vi "Error Check.vi"(8 "error in":errorcluster, 10 "Error Query Command":string, 11 "VISA Interface in":refnum<class "VISA Interface.lvclass">) -> (0 "error out":errorcluster, 3 "VISA Interface out":refnum<class "VISA Interface.lvclass">)   [LabVIEW 2020, in "Plugin Instrument Driver.lvlib" / "VISA Interface.lvclass"]
doc: "This VI Sets the error query command and reads the response from instrument."
uses:
  VISA Interface.lvclass
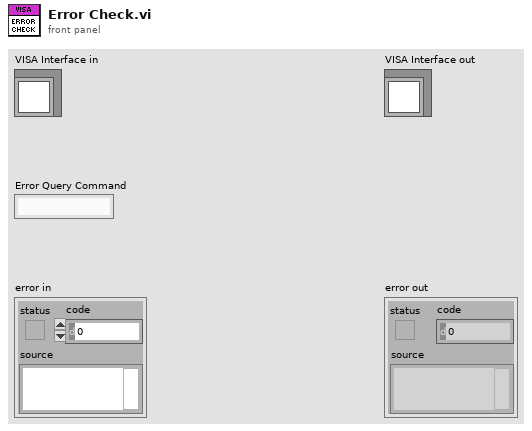
[diagram p1: front panel]
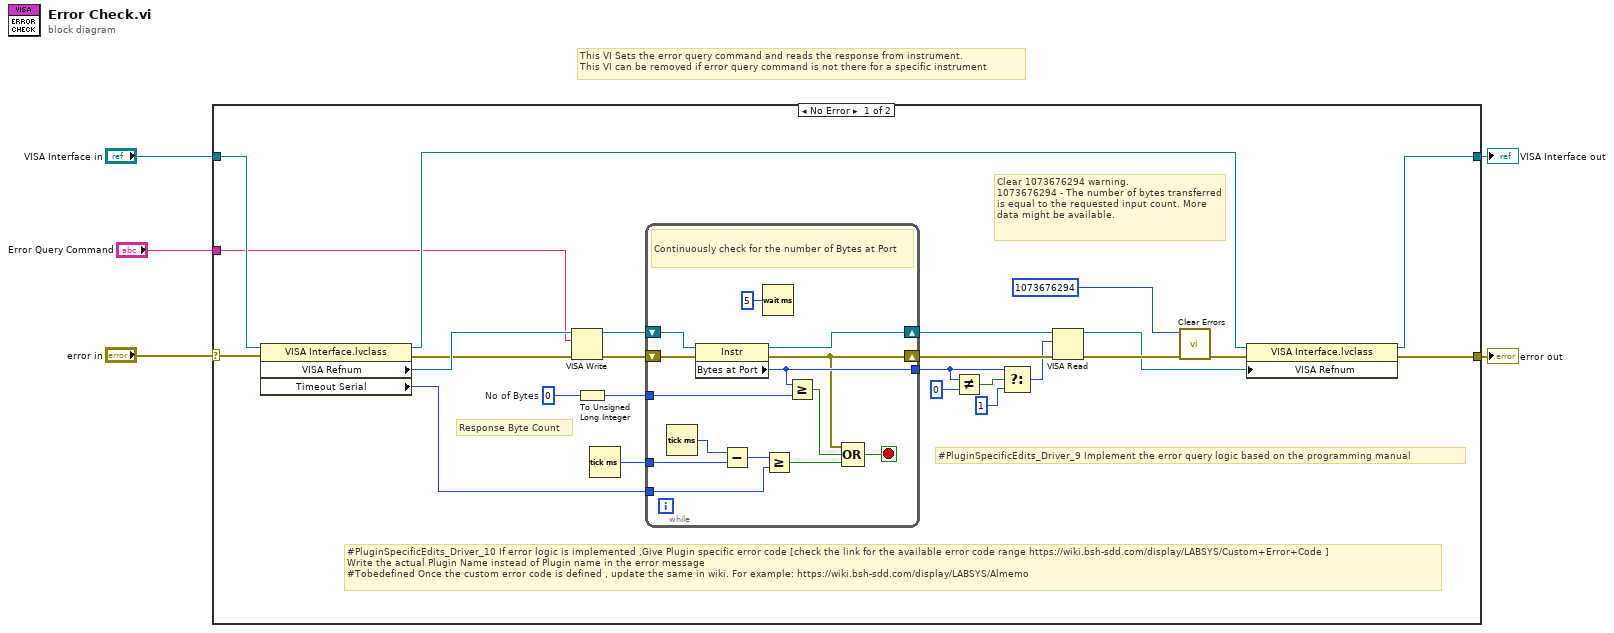
[diagram p0: block diagram]
diagram:
  # "This VI Sets the error query command and reads the response from instrument. \nThis VI can be removed if error query command is not there for a specific instrument"
  n1 = case shown="No Error" "error in" {
    selector: "error in" -> [w9 w45]
    tunnel: [w11 w46] -> w3
    tunnel: "VISA Interface in" -> [w12 w46]
    tunnel: [w10 w45] -> w2
    tunnel: "Error Query Command" -> [w6 _]
    frame No Error {
      w19 = u32 0  # No of Bytes
      # "#PluginSpecificEdits_Driver_10 If error logic is implemented ,Give Plugin specific error code [check the link for the available error code range https://wiki.bsh-sdd.com/display/LABSYS/Custom+Error+Code ]\nWrite the actual Plugin Name instead of Plugin name in the error message\n#Tobedefined Once the custom error code is defined , update the same in wiki. For example: https://wiki.bsh-sdd.com/display/LABSYS/Almemo"
      # "#PluginSpecificEdits_Driver_9 Implement the error query logic based on the programming manual"
      # "Clear 1073676294 warning.\n1073676294 - The number of bytes transferred is equal to the requested input count. More data might be available."
      # "Response Byte Count"
      n2 = property class="VISA Interface.lvclass"(reference=w12, error in=w9) -> (reference out=w15:refnum<class "VISA Interface.lvclass">, error out=w7:errorcluster, "VISA Refnum"=w8:refnum<visa-resource-name>, "Timeout Serial"=w18:u32)
      n3 = VISA Write(VISA resource name=w8, write buffer=w6, error in (no error)=w7) -> (VISA resource name out=w28:refnum<visa-resource-name>, error out=w30:errorcluster)  [unwired: 1 out]
      n4 = To Unsigned Long Integer(number=w19) -> (unsigned 32bit integer=w25:u32)
      n5 = Tick Count (ms)() -> (millisecond timer value=w26:u32)
      n6 = while {
        tunnel: [w41] -> w20
        shift-right: [w36] -> w29
        shift-left: w30 -> [w44]
        shift-right: [w42] -> w27
        shift-left: w28 -> [w43]
        tunnel: w26 -> [w38]
        tunnel: w25 -> [w32]
        tunnel: w18 -> [w31]
        stop <- w33 stop-if-true
        # "Continuously check for the number of Bytes at Port"
        n7 = Tick Count (ms)() -> (millisecond timer value=w39:u32)
        n8 = property class="Instr"(reference=w43, error in=w44) -> (reference out=w42:refnum<visa-resource-name>, error out=w36:errorcluster, "Bytes at Port"=w41:u32)
        n9 = Subtract(x=w39, y=w38) -> (x-y=w37:u32)
        n10 = Wait (ms)(milliseconds to wait=u32 5) -> ()  [unwired: 1 out]
        n11 = Greater Or Equal?(x=w37, y=w31) -> (x >= y?=w34:bool)
        n12 = Greater Or Equal?(x=w41, y=w32) -> (x >= y?=w35:bool)
        n13 = Compound Arithmetic op=OR(w36, w35, w34) -> (w33:bool)
      }
      n14 = Not Equal?(x=w20, y=u32 0) -> (x != y?=w23:bool)
      n15 = Select(t=w20, s=w23, f=u32 1 ("t")) -> (s? t:f=w22:u32)
      n16 = VISA Read(VISA resource name=w27, byte count=w22, error in (no error)=w29) -> (VISA resource name out=w13:refnum<visa-resource-name>, error out=w16:errorcluster)  [unwired: 2 out]
      n17 = call <vilib>:"Clear Errors.vi"("error in (no error)"=w16, "specific error code to clear (0: all)"=1073676294) -> ("error out"=w14:errorcluster)  [unwired: 4 in, 1 out]
      n18 = property class="VISA Interface.lvclass"(reference=w15, error in=w14, "VISA Refnum"=w13) -> (reference out=w11:refnum<class "VISA Interface.lvclass">, error out=w10:errorcluster)
    }
    frame Error {
    }
  }
  "error out" <- w2
  "VISA Interface out" <- w3
